vi "Get All Property Data.vi"(8 "error in":errorcluster, 11 "Item Ref in":refnum<data-value>) -> (0 "error out":errorcluster, 2 "Properties Data":T2(array[cluster]), 3 "Item Ref out":refnum<data-value>)   [LabVIEW 2024, in "Config File Parser.lvlib" / "Property.lvclass"]
uses:
  Property.lvclass
  Item/Item.lvclass
  Property Type.ctl
  Property.lvclass/Property.ctl
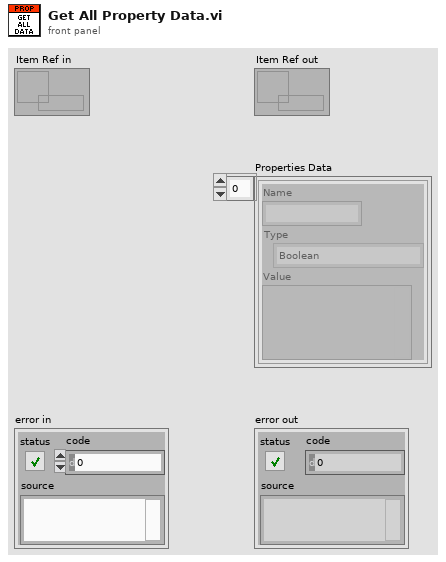
[diagram p1: front panel]
types:
  T1 = typedef "Config File Parser.lvlib/Property.lvclass/Property Type.ctl" = enum16{"Boolean", "Double", "String", "Path", "Dictionary", "DependentFile", "I16", "I32", "I64", "U16", "U32", "U64", "BooleanArray", "DoubleArray", "StringArray", "I16Array", "I32Array", "I64Array", "U16Array", "U32Array", "U64Array", "Variant"}
  T2 = cluster{"Name":string, "Type":T1, "Value":variant}[]
  T3 = cluster{"Name":string, "Type":T1, "Value":variant}
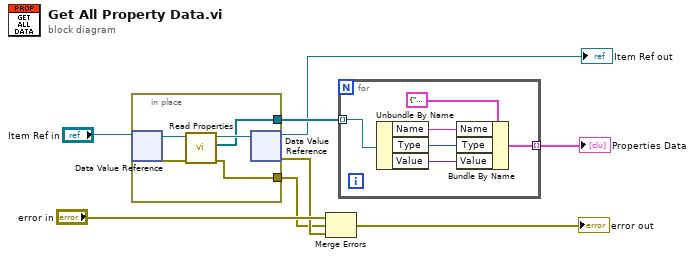
[diagram p0: block diagram]
diagram:
  n1 = in-place "In Place Element Structure" {
    in-place-border: [w12] -> w5
    in-place-border: [w9] -> w3
    n2 = in-place-dvr #1("Item Ref in") -> (w11:refnum<class "Item.lvclass">, w13:errorcluster)
    n3 = call-dynamic "Read Properties.vi"("error in (no error)"=w13, "Item in"=w11) -> ("error out"=w12:errorcluster, "Properties"=w9:refnum<class "Property.lvclass">[], "Item out"=w10:refnum<class "Item.lvclass">)  [unwired: 7 in]
    n4 = in-place-dvr #1(w10) -> (→"Item Ref out":refnum<data-value>, w7:errorcluster)
  }
  n5 = Merge Errors("error in", w5, w7) -> (→"error out":errorcluster)
  n6 = for {
    tunnel: w3 -> [w19] mode=indexing
    tunnel: [w14] -> w2 mode=indexing
    n7 = Unbundle By Name(w19) -> ("Name"=w18:string, "Type"=w16:T1, "Value"=w15:variant)
    n8 = Bundle By Name(cluster=T3 {"Name"="", "Type"=enum."Boolean", "Value"=variant}, "Name"=w18, "Type"=w16, "Value"=w15) -> (w14:T3)
  }
  "Properties Data" <- w2
